vi "pmu_Check Physical Channel Phase.vi"(8 "error in (no error)":errorcluster, 11 "physical channels in":T3[](array[typedef])) -> (0 "error out":errorcluster, 3 "physical channel out":T2(array[cluster]))   [LabVIEW 2014, in "NI_EP_PMU.lvlib"]
uses:
  <vilib>/addons/Electrical Power/PMU/NI_EP_PMU.lvlib
  <vilib>/addons/Electrical Power/PMU/Common/Controls/pmu_Physical Channel.ctl
  <vilib>/addons/Electrical Power/PMU/Common/Controls/pmu_Channel Phase.ctl
  <vilib>/addons/Electrical Power/PMU/Common/Controls/pmu_Connection Type.ctl
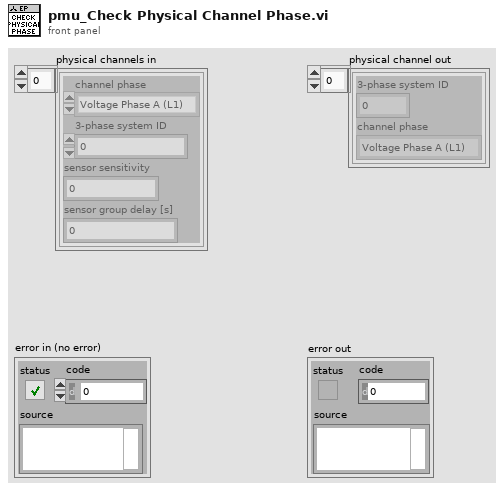
[diagram p1: front panel]
types:
  T1 = typedef "NI_EP_PMU.lvlib/pmu_Channel Phase.ctl" = enum16{"Voltage Phase A (L1)", "Voltage Phase B (L2)", "Voltage Phase C (L3)", "Voltage Phase N (Neutral)", "Current Phase A (L1)", "Current Phase B (L2)", "Current Phase C (L3)", "Current Phase N (Neutral)", "Voltage Phase AB (L1L2)", "Voltage Phase BC (L2L3)", "Voltage Phase CA (L3L1)"}
  T2 = cluster{"3-phase system ID":u8, "channel phase":T1}[]
  T3 = typedef "NI_EP_PMU.lvlib/pmu_Physical Channel.ctl" = cluster{"channel phase":T1, "3-phase system ID":u8, "sensor sensitivity":dbl, "sensor group delay [s]":dbl}
  T4 = typedef "NI_EP_PMU.lvlib/pmu_Connection Type.ctl" = enum16{"Wye", "Delta"}
  T5 = cluster{"3-phase system ID":u8, "connection type":T4}[]
  T6 = cluster{"channel phase system":u8, "channel phase":T1}[]
  T7 = cluster{"3-phase system ID":u8, "channel phase":T1}
  T8 = cluster{"3-phase system ID":u8, "connection type":T4}
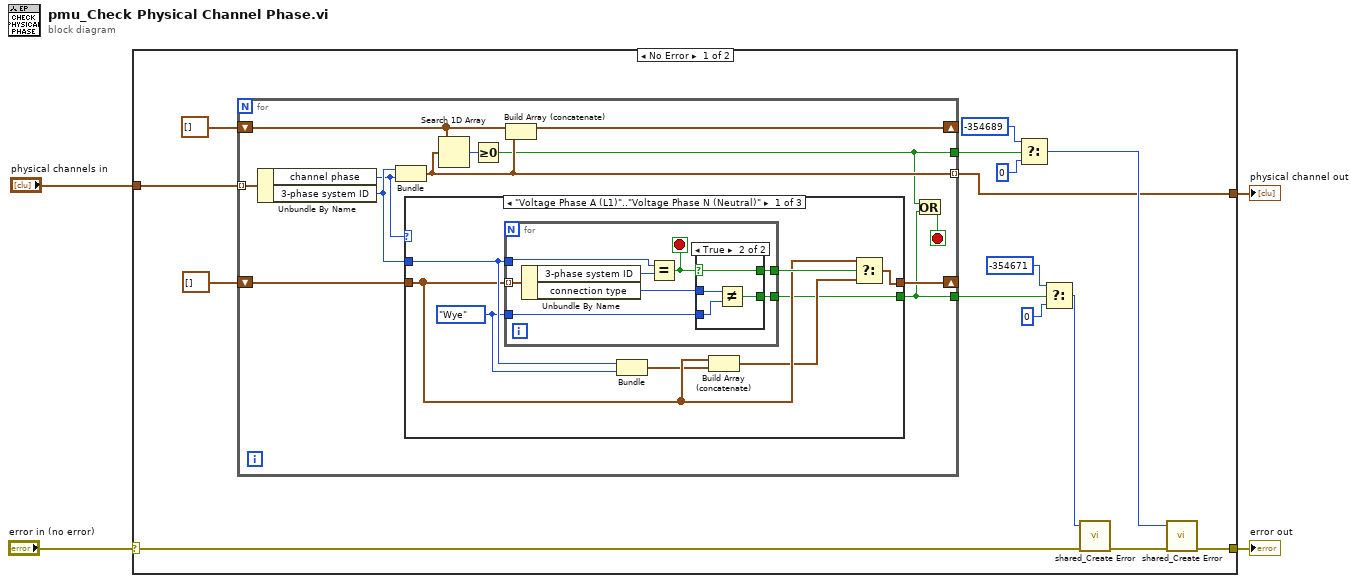
[diagram p0: block diagram]
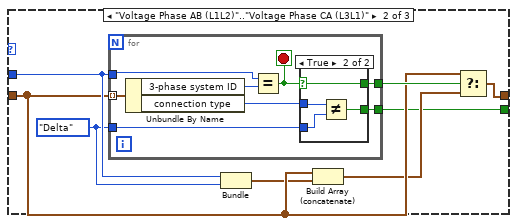
[diagram p3: hidden frame]
diagram:
  n1 = case shown="No Error" "error in (no error)" {
    selector: "error in (no error)" -> [w8 w75]
    tunnel: "physical channels in" -> [w18 _]
    tunnel: [w14 w75] -> w1
    tunnel: [w13 _] -> w2
    frame No Error {
      n2 = for {
        tunnel: w18 -> [w27] mode=indexing
        tunnel: [w29] -> w13 mode=indexing
        shift-right: [w31] -> _
        shift-left: T6 [] -> [w30]
        tunnel: [w22] -> w6
        shift-right: [w23] -> _
        shift-left: T5 [] -> [w26]
        tunnel: [w21] -> w5
        stop <- w20 stop-if-true
        n3 = Unbundle By Name(w27) -> ("channel phase"=w24:T1, "3-phase system ID"=w25:u8)
        n4 = Bundle("3-phase system ID"=w25, "channel phase"=w24) -> (w29:T7)  [unwired: 1 in]
        n5 = case shown="\"Voltage Phase A (L1)\"..\"Voltage Phase N (Neutral)\"" w24 {
          tunnel: w26 -> [w36 w57 w74]
          tunnel: w25 -> [w38 w59 _]
          tunnel: [w33 w54 w74] -> w23
          tunnel: [w32 w53 _] -> w21
          frame "Voltage Phase A (L1)".."Voltage Phase N (Neutral)" {
            w37 = pmu_Connection_Type."Wye" ("connection type")
            n6 = for {
              tunnel: w36 -> [w47] mode=indexing
              tunnel: w38 -> [w45]
              tunnel: w37 -> [w44]
              tunnel: [w41] -> w39
              tunnel: [w40] -> w32
              stop <- w42 stop-if-true
              n7 = Unbundle By Name(w47) -> ("3-phase system ID"=w46:u8, "connection type"=w43:T4)
              n8 = Equal?(x=w45, y=w46) -> (x = y?=w42:bool)
              n9 = case shown="True" w42 {
                selector: w42 -> [w48 w50]
                tunnel: w44 -> [_ w51]
                tunnel: w43 -> [_ w52]
                tunnel: [w48 w50] -> w41
                tunnel: [_ w49] -> w40
                frame False {
                }
                frame True {
                  n10 = Not Equal?(x=w52, y=w51) -> (x != y?=w49:bool)
                }
              }
            }
            n11 = Bundle("3-phase system ID"=w38, "connection type"=w37) -> (w35:T8)  [unwired: 1 in]
            n12 = Build Array (concatenate)(w36, w35) -> (w34:T5)
            n13 = Select(t=w36, s=w39, f=w34) -> (s? t:f=w33:T5)
          }
          frame "Voltage Phase AB (L1L2)".."Voltage Phase CA (L3L1)" {
            w58 = pmu_Connection_Type."Delta" ("connection type")
            n14 = for {
              tunnel: w57 -> [w68] mode=indexing
              tunnel: w59 -> [w66]
              tunnel: w58 -> [w65]
              tunnel: [w62] -> w60
              tunnel: [w61] -> w53
              stop <- w63 stop-if-true
              n15 = Unbundle By Name(w68) -> ("3-phase system ID"=w67:u8, "connection type"=w64:T4)
              n16 = Equal?(x=w66, y=w67) -> (x = y?=w63:bool)
              n17 = case shown="True" w63 {
                selector: w63 -> [w69 w71]
                tunnel: w65 -> [_ w72]
                tunnel: w64 -> [_ w73]
                tunnel: [w69 w71] -> w62
                tunnel: [_ w70] -> w61
                frame False {
                }
                frame True {
                  n18 = Not Equal?(x=w73, y=w72) -> (x != y?=w70:bool)
                }
              }
            }
            n19 = Bundle("3-phase system ID"=w59, "connection type"=w58) -> (w56:T8)  [unwired: 1 in]
            n20 = Build Array (concatenate)(w57, w56) -> (w55:T5)
            n21 = Select(t=w57, s=w60, f=w55) -> (s? t:f=w54:T5)
          }
          frame "Current Phase A (L1)".."Current Phase N (Neutral)", Default {
          }
        }
        n22 = Search 1D Array(1D array=w30, element=w29) -> (index of element=w28:i32)  [unwired: 1 in]
        n23 = Greater Or Equal To 0?(x=w28) -> (x >= 0?=w22:bool)
        n24 = Build Array (concatenate)(w30, w29) -> (w31:T2)
        n25 = Or(x=w22, y=w21) -> (x .or. y?=w20:bool)
      }
      n26 = Select(t=-354689 ("error code (0)"), s=w6, f=0 ("error code (0)")) -> (s? t:f=w15:i32)
      n27 = Select(t=-354671 ("error code (0)"), s=w5, f=0 ("error code (0)")) -> (s? t:f=w7:i32)
      n28 = call <vilib>:"shared_Create Error.vi"("error in (no error)"=w8, "error code (0)"=w7) -> ("error out"=w9:errorcluster)  [unwired: 9 in]
      n29 = call <vilib>:"shared_Create Error.vi"("error in (no error)"=w9, "error code (0)"=w15) -> ("error out"=w14:errorcluster)  [unwired: 9 in]
    }
    frame Error {
    }
  }
  "error out" <- w1
  "physical channel out" <- w2
